vi "XYStage.KIM101.OnMoveAbsolute (counts).vi"(8 "error in (no error)":errorcluster, 10 "MoveAbsolute (counts)":T1, 11 "XYStage.KIM101 in":refnum<class "XYStage.KIM101.lvclass">) -> (0 "error out":errorcluster, 3 "XYStage.KIM101 out":refnum<class "XYStage.KIM101.lvclass">)   [LabVIEW 2017, in "XYStage.KIM101.lvclass"]
uses:
  XYStage.KIM101.lvclass
  Typedefs/PrivateEvents--XYStage.KIM101.MoveAbsolute (counts).ctl
  XYStage/Typedefs/Coordinates.Counts--Cluster.ctl
  XYStage.KIM101.lvclass/XYStage.KIM101.ctl
  XYStage/XYStage.lvclass
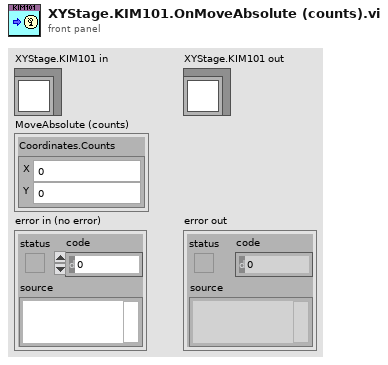
[diagram p1: front panel]
types:
  T1 = typedef "XYStage.KIM101.lvclass/PrivateEvents--XYStage.KIM101.MoveAbsolute (counts).ctl" = cluster{"Coordinates.Counts":T2}
  T2 = typedef "XYStage.lvclass/Coordinates.Counts--Cluster.ctl" = cluster{"X":i32, "Y":i32}
  T3 = typedef "XYStage.KIM101.lvclass/PrivateData--Ref.ctl" = refnum<data-value>
  T4 = typedef "XYStage.KIM101.lvclass/PrivateData--Cluster.ctl" = cluster{"Resource":T5, "Private Events":T6}
  T5 = typedef "XYStage.KIM101.lvclass/Resource--Cluster.ctl" = cluster{"KCubeInertialMotorControl":refnum<k24>, "Device":refnum<k24>, "X Axis Channel":i32, "Y Axis Channel":i32}
  T6 = typedef "XYStage.KIM101.lvclass/PrivateEvents--Cluster.ctl" = cluster{"MoveAbsolute (counts)":refnum<user-event>}
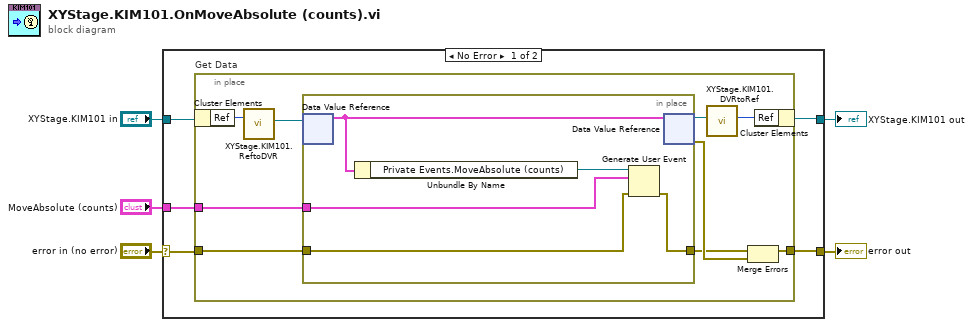
[diagram p0: block diagram]
diagram:
  n1 = case shown="No Error" "error in (no error)" {
    selector: "error in (no error)" -> [w8 w26]
    tunnel: [w7 w26] -> w4
    tunnel: [w9 w25] -> w2
    tunnel: "XYStage.KIM101 in" -> [w10 w25]
    tunnel: "MoveAbsolute (counts)" -> [w6 _]
    frame No Error {
      n2 = in-place "Get Data" {
        in-place-border: w8 -> [w19]
        in-place-border: [w16] -> w7
        in-place-border: w6 -> [w11]
        n3 = in-place-cluster #1(w10) -> ("Ref"=w15:u32)
        n4 = call "XYStage.KIM101.ReftoDVR.vi"("Ref"=w15) -> ("Ref"=w14:T3)  [unwired: 10 in]
        n5 = in-place {
          in-place-border: w19 -> [w21]
          in-place-border: [w20] -> w17
          in-place-border: w11 -> [w22]
          n6 = in-place-dvr #2(w14) -> (w24:T4)  [unwired: 1 out]
          n7 = Unbundle By Name(w24) -> ("Private Events.MoveAbsolute (counts)"=w23:refnum<user-event>)
          n8 = Generate User Event(user event=w23, event data cluster=w22, error in=w21) -> (error out=w20:errorcluster)  [unwired: 1 in, 1 out]
          n9 = in-place-dvr #2(w24) -> (w12:T3, w18:errorcluster)
        }
        n10 = call "XYStage.KIM101.DVRtoRef.vi"("Ref"=w12) -> ("Ref"=w13:u32)  [unwired: 10 in]
        n11 = Merge Errors(w17, w18) -> (w16:errorcluster)
        n12 = in-place-cluster #1("Ref"=w13) -> (w9:refnum<class "XYStage.KIM101.lvclass">)
      }
    }
    frame Error {
    }
  }
  "error out" <- w4
  "XYStage.KIM101 out" <- w2
